vi "Read OOB TX.vi"(8 "error in (no error)":errorcluster, 11 "CIFCorePlugin in":refnum<class "CIFCorePlugin.lvclass">) -> (0 "error out":errorcluster, 3 "CIFCorePlugin out":refnum<class "CIFCorePlugin.lvclass">)   [LabVIEW 2021, in "CIFCorePlugin.lvclass"]
uses:
  CIFCorePlugin.lvclass
  CIFCorePlugin.lvclass/CIFCorePlugin.ctl
  CIFUtilities/CIFOutOfBand/CIFOutOfBand.lvclass/CIFOutOfBand.ctl
  CIFUtilities/CIFChannelMng/CIFChannelMng.lvclass/CIFChannelMng.ctl
  CIFUtilities/CIFOutOfBand/Read OOB DVR.vi
  OOB/OOB_Tx/Private/Command Settings.vi
  OOB/OOB_Tx/Private/Read Payload.vi
  CIFUtilities/CIFChannelMng/Accessors/Write Channel Status for OOB.vi
  CIFUtilities/CIFOutOfBand/Accessors/Read Local OOB Data.vi
  OOB/OOB_Tx/CIFCoreOOB_Tx.lvclass
  D:/dev/CIF-LVCore/src/CIFUtilities/CIFOutOfBand/CIFOutOfBand.lvclass
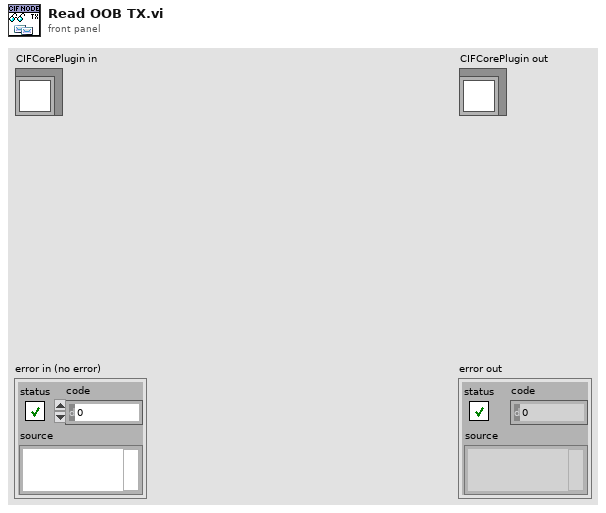
[diagram p1: front panel]
types:
  T1 = typedef "CIFCoreOOB_Tx.lvclass/OOB Core Commands.ctl" = enum8{"Status", "Overrides", "Channel List"}
  T2 = typedef "CIFCoreCommon.lvlib/Plugin Overrides.ctl" = cluster{"Timing Overrides":T3}
  T3 = typedef "CIFCoreCommon.lvlib/Timing Overrides.ctl" = cluster{"Override Timing":bool, "Skip Sleep":bool, "Period (s)":dbl}
  T4 = typedef "CIFCoreCommon.lvlib/Plugin Status.ctl" = cluster{"State":T5, "Timing Statistics (us)":T6, "FIFO Statistics (us)":T8, "error":T9, "Monitor Doubles":T10, "Monitor U64":T11, "Monitor I64":T12, "Cleanup":T7, "Create":i32, "Destroy":i32}
  T5 = typedef "CIFCoreCommon.lvlib/Plugin State.ctl" = enum32{"Null", "Creating", "Listening", "Running", "CleaningUp", "Destroying"}
  T6 = typedef "CIFCoreCommon.lvlib/Timing Statistics.ctl" = cluster{"Period":T7, "Wake Error":T7, "Execute":T7, "Housekeep":T7, "Idle":T7}
  T7 = typedef "CIFCoreCommon.lvlib/Timing Stats Base.ctl" = cluster{"Max":i32, "Min":i32}
  T8 = typedef "CIFCoreCommon.lvlib/FIFO Statistics.ctl" = cluster{"From T0":T7, "From Previous Plugin":T7, "Output Error":T7}
  T9 = typedef "CIFCoreCommon.lvlib/Simple Error.ctl" = cluster{"status":bool, "code":i32}
  T10 = typedef "CIFCoreCommon.lvlib/Monitor Doubles.ctl" = cluster{"1":dbl, "2":dbl, "3":dbl, "4":dbl}
  T11 = typedef "CIFCoreCommon.lvlib/Monitor U64.ctl" = cluster{"1":u64, "2":u64, "3":u64, "4":u64}
  T12 = typedef "CIFCoreCommon.lvlib/Monitor I64.ctl" = cluster{"1":i64, "2":i64, "3":i64, "4":i64}
  T13 = typedef "CIFChannelMng.lvclass/Channel List for OOB.ctl" = cluster{"Name":string, "Direction":T14, "Type":string, "Connected?":bool, "Connected Name":string, "Custom Config Data":u8[]}
  T14 = typedef "CIFChannels.lvclass/Direction.ctl" = enum16{"Publisher", "Subscriber"}
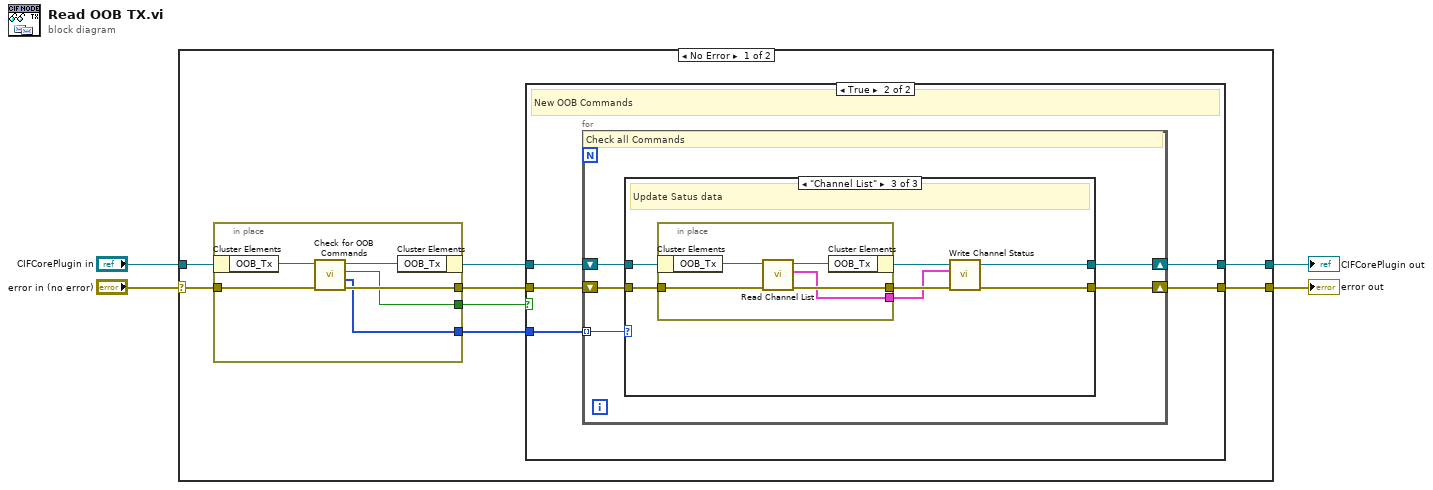
[diagram p0: block diagram]
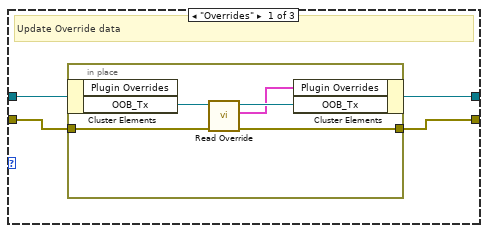
[diagram p3: hidden frame]
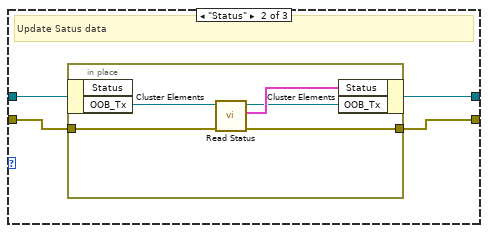
[diagram p4: hidden frame]
diagram:
  n1 = case shown="No Error" "error in (no error)" {
    selector: "error in (no error)" -> [w11 w62]
    tunnel: [w5 w62] -> w3
    tunnel: [w7 w61] -> w1
    tunnel: "CIFCorePlugin in" -> [w12 w61]
    frame No Error {
      n2 = in-place {
        in-place-border: w11 -> [w59]
        in-place-border: [w57] -> w6
        in-place-border: [w56] -> w9
        in-place-border: [w55] -> w10
        n3 = in-place-cluster #1(w12) -> ("OOB_Tx"=w60:refnum<class "CIFCoreOOB_Tx.lvclass">)
        n4 = call "Check for OOB Commands.vi"("error in (no error)"=w59, "CoreOOB_Tx in"=w60) -> ("error out"=w57:errorcluster, "Commands"=w56:T1[], "New Commands"=w55:bool, "CoreOOB_Tx out"=w58:refnum<class "CIFCoreOOB_Tx.lvclass">)  [unwired: 6 in]
        n5 = in-place-cluster #1("OOB_Tx"=w58) -> (w8:refnum<class "CIFCorePlugin.lvclass">)
      }
      n6 = case shown="True" w10 {
        tunnel: w9 -> [_ w19]
        tunnel: w8 -> [w14 w18]
        tunnel: [w14 w16] -> w7
        tunnel: w6 -> [w13 w17]
        tunnel: [w13 w15] -> w5
        frame False {
          # "No new OOB Commands"
        }
        frame True {
          # "New OOB Commands"
          n7 = for {
            tunnel: w19 -> [w24] mode=indexing
            shift-right: [w21] -> w16
            shift-left: w18 -> [w22]
            shift-right: [w20] -> w15
            shift-left: w17 -> [w23]
            # "Check all Commands"
            n8 = case shown="\"Channel List\"" w24 {
              tunnel: w23 -> [w27 w36 w49]
              tunnel: w22 -> [w28 w37 w48]
              tunnel: [w26 w35 w45] -> w21
              tunnel: [w25 w34 w44] -> w20
              frame "Overrides" {
                # "Update Override data"
                n9 = in-place {
                  in-place-border: w27 -> [w31]
                  in-place-border: [w30] -> w25
                  n10 = in-place-cluster #2(w28) -> ("OOB_Tx"=w33:refnum<class "CIFCoreOOB_Tx.lvclass">)  [unwired: 1 out]
                  n11 = call "Read Override.vi"("error in"=w31, "CoreOOB_Tx in"=w33) -> ("error out"=w30:errorcluster, "Plugin Overrides"=w29:T2, "CoreOOB_Tx out"=w32:refnum<class "CIFCoreOOB_Tx.lvclass">)  [unwired: 7 in]
                  n12 = in-place-cluster #2("Plugin Overrides"=w29, "OOB_Tx"=w32) -> (w26:refnum<class "CIFCorePlugin.lvclass">)
                }
              }
              frame "Status" {
                # "Update Satus data"
                n13 = in-place {
                  in-place-border: w36 -> [w41]
                  in-place-border: [w38] -> w34
                  n14 = in-place-cluster #3(w37) -> ("OOB_Tx"=w42:refnum<class "CIFCoreOOB_Tx.lvclass">)  [unwired: 1 out]
                  n15 = call "Read Status.vi"("error in"=w41, "CoreOOB_Tx in"=w42) -> ("error out"=w38:errorcluster, "Status"=w40:T4, "CoreOOB_Tx out"=w39:refnum<class "CIFCoreOOB_Tx.lvclass">)  [unwired: 7 in]
                  n16 = in-place-cluster #3("Status"=w40, "OOB_Tx"=w39) -> (w35:refnum<class "CIFCorePlugin.lvclass">)
                }
              }
              frame "Channel List" {
                # "Update Satus data"
                n17 = in-place {
                  in-place-border: w49 -> [w53]
                  in-place-border: [w51] -> w46
                  in-place-border: [w50] -> w43
                  n18 = in-place-cluster #4(w48) -> ("OOB_Tx"=w54:refnum<class "CIFCoreOOB_Tx.lvclass">)
                  n19 = call "Read Channel List.vi"("error in"=w53, "CoreOOB_Tx in"=w54) -> ("error out"=w51:errorcluster, "Channel List"=w50:T13[], "CoreOOB_Tx out"=w52:refnum<class "CIFCoreOOB_Tx.lvclass">)  [unwired: 7 in]
                  n20 = in-place-cluster #4("OOB_Tx"=w52) -> (w47:refnum<class "CIFCorePlugin.lvclass">)
                }
                n21 = call "Write Channel Status.vi"("error in (no error)"=w46, "Channel Status"=w43, "CIFCorePlugin in"=w47) -> ("error out"=w44:errorcluster, "CIFCorePlugin out"=w45:refnum<class "CIFCorePlugin.lvclass">)  [unwired: 7 in]
              }
            }
          }
        }
      }
    }
    frame Error {
    }
  }
  "error out" <- w3
  "CIFCorePlugin out" <- w1
